vi "PC_name.vi"() -> (0 "this computer's name":string)   [LabVIEW 2015]
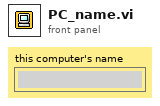
[diagram p1: front panel]
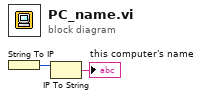
[diagram p0: block diagram]
diagram:
  n1 = String To IP() -> (0:w2:u32)  [unwired: 1 in]
  n2 = IP To String(2:w2) -> (0:→"this computer's name":string)  [unwired: 1 in]
